vi "Read from DB.vi"(8 "error in (no error)":errorcluster) -> (0 "error out":errorcluster, 2 "Array":T1[](array[typedef]) {"Balance" format="%.2f"; "Account" format="%05d"}, 3 "refnum out":refnum<file>)   [LabVIEW 2017]
uses:
  Type Definitions/DB Record.ctl
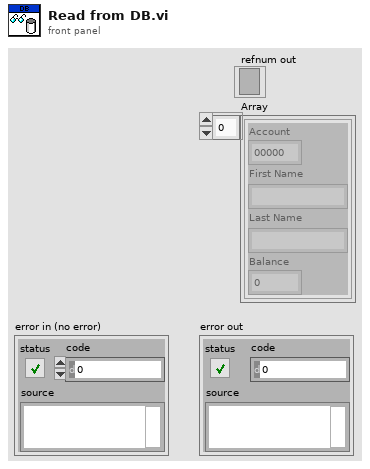
[diagram p1: front panel]
types:
  T1 = typedef "DB Record.ctl" = cluster{"Account":i32, "First Name":string, "Last Name":string, "Balance":fxp<+/-,64,35>}
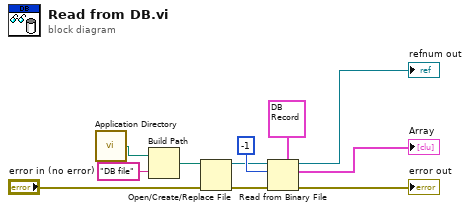
[diagram p0: block diagram]
diagram:
  n1 = call <vilib>:"Application Directory.vi"() -> ("Application Directory"=w2:path)
  n2 = Build Path(base path=w2, name or relative path="DB file") -> (appended path=w4:path)
  n3 = Open/Create/Replace File(file path (use dialog)=w4, error in="error in (no error)") -> (refnum out=w5:refnum<file>, error out=w8:errorcluster)  [unwired: 4 in, 1 out]
  n4 = Read from Binary File(5:T1 {"Account"=0, "First Name"="", "Last Name"="", "Balance"=0.0} ("DB Record"), 8:w8, 10:-1 ("count (1)"), 11:w5) -> (0:→"error out":errorcluster, 2:→"Array":T1[], 3:→"refnum out":refnum<file>)  [unwired: 2 in, 1 out]
